vi "Write Vars.vi"(8 "error in (no error)":errorcluster, 10 "Vars":refnum<class "Abs_Value.lvclass">[](array[class]), 11 "Local Vars in":refnum<class "Local Vars.lvclass">) -> (0 "error out":errorcluster, 3 "Local Vars out":refnum<class "Local Vars.lvclass">)   [LabVIEW 2021]
uses:
  Local Vars.lvclass
  LV_Abstract/Source/Abs_Types/Value/Abs_Value.lvclass
  Local Vars.lvclass/Local Vars.ctl
  C:/Users/Tim/Documents/GitHub/VarBus/Source/Var Access/Var_Access.lvclass
  C:/Users/Tim/Documents/GitHub/LV_Abstract/Source/Abs_Types/Type/Abs_Type.lvclass
  C:/Users/Tim/Documents/GitHub/VarBus/Source/Local Vars/Local Vars.lvclass
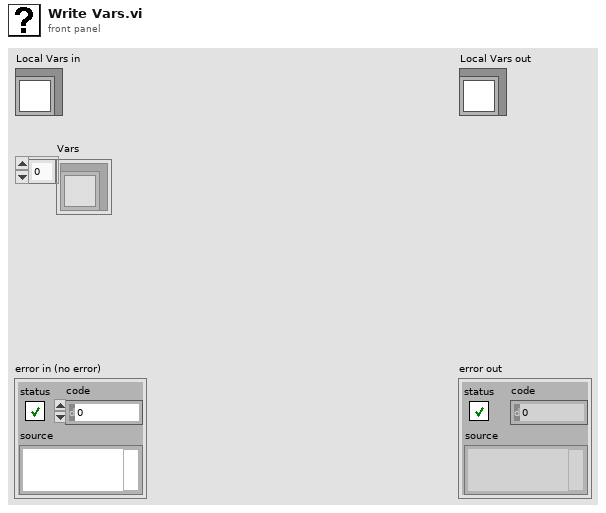
[diagram p1: front panel]
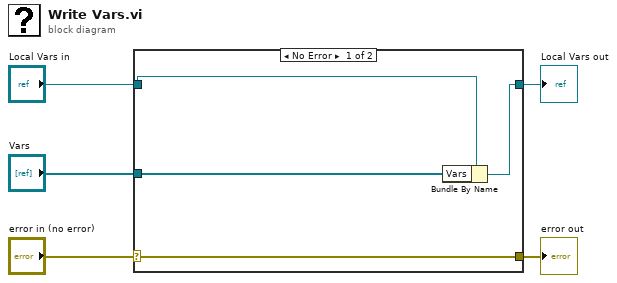
[diagram p0: block diagram]
diagram:
  n1 = case shown="No Error" "error in (no error)" {
    selector: "error in (no error)" -> [w9 w10]
    tunnel: [w9 w10] -> w4
    tunnel: [w7 w11] -> w2
    tunnel: "Local Vars in" -> [w8 w11]
    tunnel: "Vars" -> [w6 _]
    frame No Error {
      n2 = Bundle By Name(cluster=w8, "Vars"=w6) -> (w7:refnum<class "Local Vars.lvclass">)
    }
    frame Error {
    }
  }
  "error out" <- w4
  "Local Vars out" <- w2
